vi "Example.vi"() -> ()   [LabVIEW 2013, in "Mercury iXX.lvlib"]
uses:
  <instrlib>/Mercury iXX/Mercury iXX.lvlib
  <instrlib>/Mercury iXX/Public/Controls/Unit String.ctl
  <instrlib>/Mercury iXX/Public/Libraries/Temperature/Controls/Temperature Device (Read).ctl
  <instrlib>/Mercury iXX/Public/Controls/Manufacturing Data.ctl
  <instrlib>/Mercury iXX/Public/Libraries/Temperature/Controls/Temperature Sensor Type.ctl
  <instrlib>/Mercury iXX/Public/Libraries/Temperature/Controls/Excitation Cluster.ctl
  <instrlib>/Mercury iXX/Public/Libraries/Temperature/Controls/Excitation Type.ctl
  <instrlib>/Mercury iXX/Public/Libraries/Temperature/Controls/Calibration Cluster.ctl
  <instrlib>/Mercury iXX/Public/Libraries/Temperature/Controls/Calibration Interpolation.ctl
  <instrlib>/Mercury iXX/Public/Libraries/Temperature/Controls/Loop Cluster.ctl
  <instrlib>/Mercury iXX/Public/Libraries/Temperature/Controls/Temperature Signals Cluster.ctl
  <instrlib>/Mercury iXX/Public/Libraries/Heater/Controls/Heater Device (Read).ctl
  <instrlib>/Mercury iXX/Public/Libraries/Heater/Controls/Heater Signals Cluster.ctl
  <instrlib>/Mercury iXX/Public/Libraries/Level Meter/Controls/Level Meter (Read).ctl
  <instrlib>/Mercury iXX/Public/Libraries/Level Meter/Controls/Nitrogen Configuration.ctl
  <instrlib>/Mercury iXX/Public/Libraries/Level Meter/Controls/Frequency Configuration.ctl
  <instrlib>/Mercury iXX/Public/Libraries/Level Meter/Controls/Signals.ctl
  <instrlib>/Mercury iXX/Public/Libraries/Level Meter/Controls/Helium Configuration.ctl
  <instrlib>/Mercury iXX/Public/Libraries/Level Meter/Controls/Resistance Configuration.ctl
  <instrlib>/Mercury iXX/Public/Libraries/Level Meter/Controls/Pre-Pulse.ctl
  <instrlib>/Mercury iXX/Public/Libraries/Level Meter/Controls/Pulse.ctl
  <instrlib>/Mercury iXX/Public/Libraries/Auxiliary/Controls/AUX Device (Read).ctl
  <instrlib>/Mercury iXX/Public/Libraries/Auxiliary/Controls/AUX Signals (Read).ctl
  <instrlib>/Mercury iXX/Public/Libraries/Magnet/Controls/Device (Read).ctl
  <instrlib>/Mercury iXX/Public/Libraries/Magnet/Controls/Signals (Read).ctl
  <instrlib>/Mercury iXX/Public/Libraries/Magnet/Controls/Identifier.ctl
  <instrlib>/Mercury iXX/Public/Libraries/Flow/Controls/Flow Device (Read).ctl
  <instrlib>/Mercury iXX/Public/Libraries/Flow/Controls/Flow Signals Cluster.ctl
  <instrlib>/Mercury iXX/Public/Libraries/Pressure/Controls/Pressure Device (Read).ctl
  <instrlib>/Mercury iXX/Public/Libraries/Pressure/Controls/Pressure Sensor Type.ctl
  <instrlib>/Mercury iXX/Public/Libraries/Pressure/Controls/Calibration Cluster.ctl
  <instrlib>/Mercury iXX/Public/Libraries/Pressure/Controls/Calibration Interpolation.ctl
  <instrlib>/Mercury iXX/Public/Libraries/Pressure/Controls/Loop Cluster.ctl
  <instrlib>/Mercury iXX/Public/Libraries/Pressure/Controls/Pressure Signals Cluster.ctl
  <instrlib>/Mercury iXX/Public/Controls/Comms Transport Layer.ctl
  <instrlib>/Mercury iXX/Public/Controls/ISOBus Address.ctl
  <instrlib>/Mercury iXX/Public/Libraries/System/Open/Open System.vi
  <instrlib>/Mercury iXX/Public/Libraries/Pressure/Open/Open Pressure Device.vi
  <instrlib>/Mercury iXX/Public/Libraries/Pressure/Configuration/Read/Pressure Device (Read).vi
  <instrlib>/Mercury iXX/Public/Libraries/Pressure/Configuration/Read/Nickname (Read).vi
  <instrlib>/Mercury iXX/Public/Libraries/Pressure/Signals/Read/Current (Read).vi
  <instrlib>/Mercury iXX/Public/Libraries/Pressure/Signals/Read/Voltage (Read).vi
  <instrlib>/Mercury iXX/Public/Libraries/Flow/Open/Open Flow Device.vi
  <instrlib>/Mercury iXX/Public/Libraries/Flow/Configuration/Read/Flow Device (Read).vi
  <instrlib>/Mercury iXX/Public/Libraries/Flow/Configuration/Read/Maximum Power (Read).vi
  <instrlib>/Mercury iXX/Public/Libraries/Flow/Configuration/Read/Fastcool Mode (Read).vi
  <instrlib>/Mercury iXX/Public/Libraries/Flow/Signals/Read/Current (Read).vi
  <instrlib>/Mercury iXX/Public/Libraries/Flow/Signals/Read/Voltage (Read).vi
  <instrlib>/Mercury iXX/Public/Libraries/System/Read/Catalogue (Read).vi
  <instrlib>/Mercury iXX/Public/Libraries/Auxiliary/Open/Open Auxiliary Device.vi
  <instrlib>/Mercury iXX/Public/Libraries/Auxiliary/Configuration/Read/Aux Device (Read).vi
  <instrlib>/Mercury iXX/Public/Libraries/Auxiliary/Configuration/Read/Serial Number (Read).vi
  <instrlib>/Mercury iXX/Public/Libraries/Auxiliary/Configuration/Read/Minimum Gas Flow (Read).vi
  <instrlib>/Mercury iXX/Public/Libraries/Auxiliary/Configuration/Read/Gas Flow Scaling (Read).vi
  <instrlib>/Mercury iXX/Public/Libraries/Auxiliary/Configuration/Read/Temperature Error Sensitivity (Read).vi
  <instrlib>/Mercury iXX/Public/Libraries/Auxiliary/Configuration/Read/Temperature Error Voltage Sensitivity (Read).vi
  <instrlib>/Mercury iXX/Public/Libraries/Auxiliary/Configuration/Read/Valve Gearing (Read).vi
  <instrlib>/Mercury iXX/Public/Libraries/Auxiliary/Configuration/Read/Stepper Speed (Read).vi
  <instrlib>/Mercury iXX/Public/Libraries/Auxiliary/Signals/Read/Position (Read).vi
  <instrlib>/Mercury iXX/Public/Libraries/Auxiliary/Signals/Read/Percent Open (Read).vi
  <instrlib>/Mercury iXX/Public/Libraries/Level Meter/Open/Open Level Meter Device.vi
  <instrlib>/Mercury iXX/Public/Libraries/Level Meter/Configuration/Read/Level Meter Device (Read).vi
  <instrlib>/Mercury iXX/Public/Libraries/Level Meter/Configuration/Read/Serial Number (Read).vi
  <instrlib>/Mercury iXX/Public/Libraries/Level Meter/Configuration/Read/Helium Probe Resistance (Read).vi
  <instrlib>/Mercury iXX/Public/Libraries/Level Meter/Configuration/Read/Helium Pulse Mag (Read).vi
  <instrlib>/Mercury iXX/Public/Libraries/Level Meter/Configuration/Read/Helium Pulse Duration (Read).vi
  <instrlib>/Mercury iXX/Public/Libraries/Level Meter/Configuration/Read/Nitrogen Freq at 100 (Read).vi
  <instrlib>/Mercury iXX/Public/Libraries/Level Meter/Configuration/Read/Nitrogen Pulse Count Period (Read).vi
  <instrlib>/Mercury iXX/Public/Libraries/Level Meter/Signals/Read/Probe Resistance Helium (Read).vi
  <instrlib>/Mercury iXX/Public/Libraries/Level Meter/Signals/Read/Probe Level Helium (Read).vi
  <instrlib>/Mercury iXX/Public/Libraries/Level Meter/Signals/Read/Probe Count Nitrogen (Read).vi
  <instrlib>/Mercury iXX/Public/Libraries/Level Meter/Signals/Read/Probe Level Nitrogen (Read).vi
  <instrlib>/Mercury iXX/Public/Libraries/System/Read/Display Automatic Dimming (Read).vi
  <instrlib>/Mercury iXX/Public/Libraries/System/Read/Display Automatic Dimming Time (Read).vi
  <instrlib>/Mercury iXX/Public/Libraries/System/Read/Display Brightness (Read).vi
  <instrlib>/Mercury iXX/Public/Libraries/System/Read/Date (Read).vi
  <instrlib>/Mercury iXX/Public/Libraries/System/Read/Time (Read).vi
  <instrlib>/Mercury iXX/Public/Libraries/System/Read/DateTime (Read).vi
  <instrlib>/Mercury iXX/Public/Libraries/System/Read/HVer (Read).vi
  <instrlib>/Mercury iXX/Public/Libraries/System/Read/FVer (Read).vi
  <instrlib>/Mercury iXX/Public/Libraries/System/Read/Serial Number (Read).vi
  <instrlib>/Mercury iXX/Public/Libraries/System/Read/Flash Space (Read).vi
  <instrlib>/Mercury iXX/Public/Libraries/System/Read/Mode (Read).vi
  <instrlib>/Mercury iXX/Public/Libraries/Temperature/Open/Open Temperature Device.vi
  <instrlib>/Mercury iXX/Public/Libraries/Temperature/Configuration/Read/Serial Number (Read).vi
  <instrlib>/Mercury iXX/Public/Libraries/Temperature/Configuration/Read/Nickname (Read).vi
  <instrlib>/Mercury iXX/Public/Libraries/Temperature/Configuration/Read/Excitation Magnitude (Read).vi
  <instrlib>/Mercury iXX/Public/Libraries/Temperature/Configuration/Read/Temperature Sensor (Read).vi
  <instrlib>/Mercury iXX/Public/Libraries/Temperature/Configuration/Read/Excitation Type (Read).vi
  <instrlib>/Mercury iXX/Public/Libraries/Temperature/Configuration/Read/Calibration Hot Limit (Read).vi
  <instrlib>/Mercury iXX/Public/Libraries/Temperature/Configuration/Read/Calibration Cold Limit (Read).vi
  <instrlib>/Mercury iXX/Public/Libraries/Temperature/Signals/Read/Temperature (Read).vi
  <instrlib>/Mercury iXX/Public/Libraries/Temperature/Configuration/Read/Temperature Device (Read).vi
  <instrlib>/Mercury iXX/Public/Libraries/Control Loop/Configuration/Read/Control Loop (Read).vi
  <instrlib>/Mercury iXX/Public/Libraries/Heater/Open/Open Heater Device.vi
  <instrlib>/Mercury iXX/Public/Libraries/Heater/Configuration/Read/Heater Device (Read).vi
  <instrlib>/Mercury iXX/Public/Libraries/Heater/Configuration/Read/Nickname (Read).vi
  <instrlib>/Mercury iXX/Public/Libraries/Heater/Configuration/Read/Serial Number (Read).vi
  <instrlib>/Mercury iXX/Public/Libraries/Heater/Configuration/Read/Voltage Limit (Read).vi
  <instrlib>/Mercury iXX/Public/Libraries/Heater/Configuration/Read/Nominal Resistance (Read).vi
  <instrlib>/Mercury iXX/Public/Libraries/Heater/Configuration/Read/Maximum Power (Read).vi
  <instrlib>/Mercury iXX/Public/Libraries/Heater/Signals/Read/Voltage (Read).vi
  <instrlib>/Mercury iXX/Public/Libraries/Heater/Signals/Read/Power (Read).vi
  <instrlib>/Mercury iXX/Public/Libraries/Heater/Signals/Read/Current (Read).vi
  <instrlib>/Mercury iXX/Public/Libraries/System/Set/DateTime (Set).vi
  <instrlib>/Mercury iXX/Public/Libraries/Magnet/Open/Open Magnet Device.vi
  <instrlib>/Mercury iXX/Public/Libraries/Magnet/Configuration/Read/Magnet Device (Read).vi
  <instrlib>/Mercury iXX/Public/Libraries/Magnet/Configuration/Read/Serial Number (Read).vi
  <instrlib>/Mercury iXX/Public/Libraries/Magnet/Configuration/Read/Bipolar Output (Read).vi
  <instrlib>/Mercury iXX/Public/Libraries/Magnet/Configuration/Read/Output Configuration (Read).vi
  <instrlib>/Mercury iXX/Public/Libraries/Magnet/Configuration/Read/Current Limit (Read).vi
  <instrlib>/Mercury iXX/Public/Libraries/Magnet/Configuration/Read/Current to Field Factor (Read).vi
  <instrlib>/Mercury iXX/Public/Libraries/Magnet/Configuration/Read/Switch Present (Read).vi
  <instrlib>/Mercury iXX/Public/Libraries/Magnet/Configuration/Read/Software Voltage Limit (Read).vi
  <instrlib>/Mercury iXX/Public/Libraries/Magnet/Signals/Read/Current Rate (Read).vi
  <instrlib>/Mercury iXX/Public/Libraries/Magnet/Configuration/Read/PSU Action Status (Read).vi
  <instrlib>/Mercury iXX/Public/Libraries/Flow.lvlib
  <instrlib>/Mercury iXX/Public/Libraries/Pressure.lvlib
  <instrlib>/Mercury iXX/Public/Libraries/System.lvlib
  <instrlib>/Mercury iXX/Public/Libraries/Level Meter.lvlib
  <instrlib>/Mercury iXX/Public/Libraries/Magnet.lvlib
  <instrlib>/Mercury iXX/Public/Libraries/Auxiliary.lvlib
  <instrlib>/Mercury iXX/Public/Libraries/Control Loop.lvlib
  <instrlib>/Mercury iXX/Public/Libraries/Heater.lvlib
  <instrlib>/Mercury iXX/Public/Libraries/Temperature.lvlib
panel:
  in  "Mercury Functions":T1(tab)
  in  "IPS IP Address":string="130.49.180.102"
  out "time stamp":timestamp=timestamp(3542718986 s since 1904-01-01)
  out "Free Space":i32=166152 caption="Free Space (KB)"
  out "Set Date Response":string="VALID"
  out "String":string="NORM" caption="User Mode"
  out "Date":string="2016:04:05"
  out "Time":string="11:36:26"
  out "Hardware Version":string="65"
  out "Firmware Version":string="2.2.6.20"
  out "Serial Number":string="153350063"
  out "Devices":string[](array[string])=["DB3.L1:LVL", "GRPX:PSU", "GRPY:PSU", "GRPZ:PSU", "MB1.T1:TEMP", "PSU.M1:PSU", "PSU.M2:PSU", "PSU.M3:PSU"]
  out "S/W Version(s)":string[](array[string])=["2.2.6.20\n"]
  out "Serial Number(s)":string[](array[string])=["153350063"]
  out "# of Instruments":i32=1
  out "Automatic Dimming":string="OFF"
  out "Dimming Time":string="5"
  out "Display Brightness":string="100"
  in  "ITC IP Address":string="130.49.180.102"
  out "Excitation Magnitude":dbl
  out "Sensor Type":string="DUM"
  out "Excitation Type":string="UNIP"
  out "Hot Limit":dbl=1000.0
  out "H Unit":T2="K"
  out "Cold Limit":dbl=1000.0
  out "C Unit":T2="K"
  out "Unit":T2
  out "Voltage":dbl
  out "V Unit":T2="A"
  out "Temperature":dbl
  out "T Unit":T2="K"
  out "Temperature Device Settings":T3={"Manufacturing"={"Hardware Version"="65", "Firmware Version"="2.2", "Serial Number"="153350063"}, "Temperature Sensor Type"="DUM", "Excitation"={"Excitation Type"="UNIP", "Magnitude"="0"}, "Calibration"={"Filename"="None", "Interpolation"="LIN", "Scaling Factor"="1", "Offset Factor"="0", "Hot Limit"="1000.00K", "Cold Limit"="1000.00K", "Last Calibration"="", "Reference"="Internal"}, "Control Loop"={"Heater"="", "Auxiliary"="", "Heater Auto"="", "Percentage Heat"="", "Temperature Set Point"="", "PID Auto (from file)"="", "P Value"="", "I Value"="", "D Value"="", "Auto PID Table Filename"="", "Flow Auto"="", "Target Heater Table"="", "Sweep mode"="", "Sweep Table Filename"="", "Percentage Flow"=""}, "Temperature Signals"={"Voltage"="0.0000V", "Current"="0.0000A", "Power"="N/A", "Resistance"="", "Temperature"="0.0000K", "Sensitivity"="", "Reference"=""}, "Nickname"="MB1.T1", "Status"="0"}
  out "Temp S/N":string="153350063"
  out "T Nickname":string="MB1.T1"
  out "T Loop Details":T10
  out "Heater Device Settings":T12={"Manufacturing"={"Hardware Version"="", "Firmware Version"="", "Serial Number"=""}, "Nickname"="", "Voltage Limit"="", "Nominal Resistance"="", "Maximum Power"="", "Heater Signals"={"Voltage"="", "Current"="", "Power"=""}, "Status"="DEV"}
  out "Htr C Unit":T2
  out "Htr P Unit":T2
  out "Htr V Unit":T2
  out "Htr Current":dbl
  out "Htr Power":dbl
  out "Htr Voltage":dbl
  out "Power Unit":T2
  out "Volt Unit":T2
  out "Res Unit":T2
  out "Maximum Power":dbl
  out "Htr Resistance":dbl
  out "Htr Voltage Limit":dbl
  out "Htr S/N":string="STAT:DEV:MB0.H1:N/A"
  out "Htr Nickname":string="STAT:DEV:MB0.H1:N/A"
  out "LVL Device DetailSettings":T14
  out "LVL S/N":string
  out "LVL P Magnitude":dbl=-inf caption="Pulse Magnitude (mA)"
  out "LVL P Duration":dbl=-inf caption="Pulse Duration (s)"
  out "N Freq 100%":dbl=-inf caption="Frequency at 100% (Hz)"
  out "N Pulse Period":dbl=-inf caption="Pulse Period (ms)"
  out "He Res Config":T19
  out "He Resistance":dbl=-inf caption="Resistance (Ohms)"
  out "He Level":dbl=-inf caption="Helium Level (%)"
  out "N Counter":u32 caption="Counter"
  out "N Level":dbl=-inf caption="Nitrogen Level (%)"
  out "Auxiliary Device Details":T22 {"Signals"."% Open" min=0.0 max=100.0 step=0.1 format="%.4f"; "Signals"."Position" max=20.0 step=1.0 format="%.4f"; "Speed" max=7 step=1; "Gear" max=7 step=1; "Temp V Err" min=0.0 max=20.0 step=0.1; "Temp Err" min=0.0 max=20.0 step=0.1; "Scaling Factor" min=0.0 max=99.0 step=0.1; "Min Flow" min=0.0 max=20.0 step=0.1}
  out "Aux S/N":string
  out "Min Flow":dbl=-inf caption="Minimum Gas Flow" format="%#.1f"
  out "Scaling Factor":dbl=-inf caption="Gas Flow Scaling Factor" format="%#.1f"
  out "Temp Err":dbl=-inf caption="Temperature Error Sensitivity" format="%#.1f"
  out "Temp V Err":dbl=-inf caption="Temperature Voltage Error Sensitivity" format="%#.1f"
  out "Gear":u32 caption="Valve Gearing"
  out "Speed":u32 caption="Stepper Speed"
  out "Unit 2":T2="ERR"
  out "Unit 3":T2="ERR"
  out "Unit 4":T2="ERR"
  out "Unit 5":T2="ERR"
  out "Unit 6":T2="ERR"
  out "Unit 7":T2="ERR"
  out "Position":u32
  out "% Open":dbl=-inf caption="Percentage Open (%)"
  out "Unit":T2="ERR"
  out "Unit":T2="ERR"
  out "Magnet Device Details":T24={"Manufacturing"={"Hardware Version"="65", "Firmware Version"="2.4", "Serial Number"="151250009"}, "Nickname"="PSU.M1", "Bipolar Output"="ON", "String"="NOT_FOUND", "Current Limit"=58.0, "AtoB"=1.0, "Inductance"=39.406, "Switch Present"="NOT_FOUND", "Swh Htr Current"=86.0, "SW VLIM"=9.0, "V Trans Time"=1000.0, "Magnet PSU Signals"={"Voltage"=-0.0003, "Current"=0.0002, "Current Rate"=0.0, "Field"=0.0, "Field Rate"=0.0, "Persistant Current"=0.0, "Persistant Field"=0.0, "Target Current"=0.0, "Target Field"=0.0, "Target Current Rate"=0.0, "Target Field Rate"=0.0, "Switch Heater Status (SWHT)"="NOT_FOUND", "Switch Heater Status (SWHN)"="NOT_FOUND"}, "PSU Action"="NOT_FOUND", "Status"="4000", "Level Limit"=0.0, "Temperature Limit"=0.0} {"Temperature Limit" format="%#.1f"; "Level Limit" format="%#.1f"; "V Trans Time" format="%#.1f"; "SW VLIM" format="%#.1f"; "Swh Htr Current" format="%#.1f"; "Inductance" format="%#.1f"; "AtoB" format="%#.1f"; "Current Limit" format="%#.1f"}
  out "Mag S/N":string="151250009"
  out "Bipolar Output":string="ON"
  out "Out Config":string="NOT_FOUND" caption="Output Configuration"
  out "Current Limit":dbl=58.0 caption="Current Limit (A)" format="%#.1f"
  out "AtoB":dbl=1.0 caption="Current Field Factor (A/T)" format="%#.1f"
  out "Switch Present":string="NOT_FOUND"
  out "SW VLIM":dbl=9.0 caption="Software Voltage Limit (V)" format="%#.1f"
  out "Unit 8":T2
  out "Unit 9":T2
  out "Unit 10":T2
  out "Current Rate":dbl
  out "PSU Act Stat":string="NOT_FOUND" caption="PSU Action Status"
  out "Unit 11":T2
  in  "Device Identifier":T26="PSU.M1"
  in  "Magnet?":bool=TRUE
  out "Flow Device":T27={"Manufacturing"={"Hardware Version"="", "Firmware Version"="", "Serial Number"=""}, "Nickname"="", "Voltage Limit"="", "Nominal Resistance"="", "Maximum Power"="", "Flow Signals"={"Voltage"="", "Current"="", "Power"="", "Flow"=""}, "Status"="DEV", "Fastcool Mode"=""}
  out "Maximum Power":dbl
  out "Fastcool Mode":string="STAT:DEV:DB1.F1:N/A"
  out "Current":dbl
  out "Voltage":dbl
  out "Pressure Device":T29={"Manufacturing"={"Hardware Version"="", "Firmware Version"="", "Serial Number"=""}, "Temperature Sensor Type"="", "Calibration"={"Filename"="", "Interpolation"="", "Scaling Factor"="", "Offset Factor"="", "High Limit"="", "Low Limit"="", "Last Calibration"=""}, "Control Loop"={"Heater"="", "Auxiliary"="", "Heater Auto"="", "Percentage Heat"="", "Pressure Set Point"="", "PID Auto (from file)"="", "P Value"="", "I Value"="", "D Value"="", "Auto PID Table Filename"="", "Flow Auto"="", "Target Heater Table"="", "Sweep mode"="", "Sweep Table Filename"="", "Percentage Flow"=""}, "Pressure Signals"={"Voltage"="", "Current"="", "Power"="", "Pressure"=""}, "Nickname"="", "Status"="DEV"}
  out "Nickname":string="STAT:DEV:DB6.P1:N/A"
  out "Current":dbl
  out "Voltage":dbl
  # "101, 102, 67"
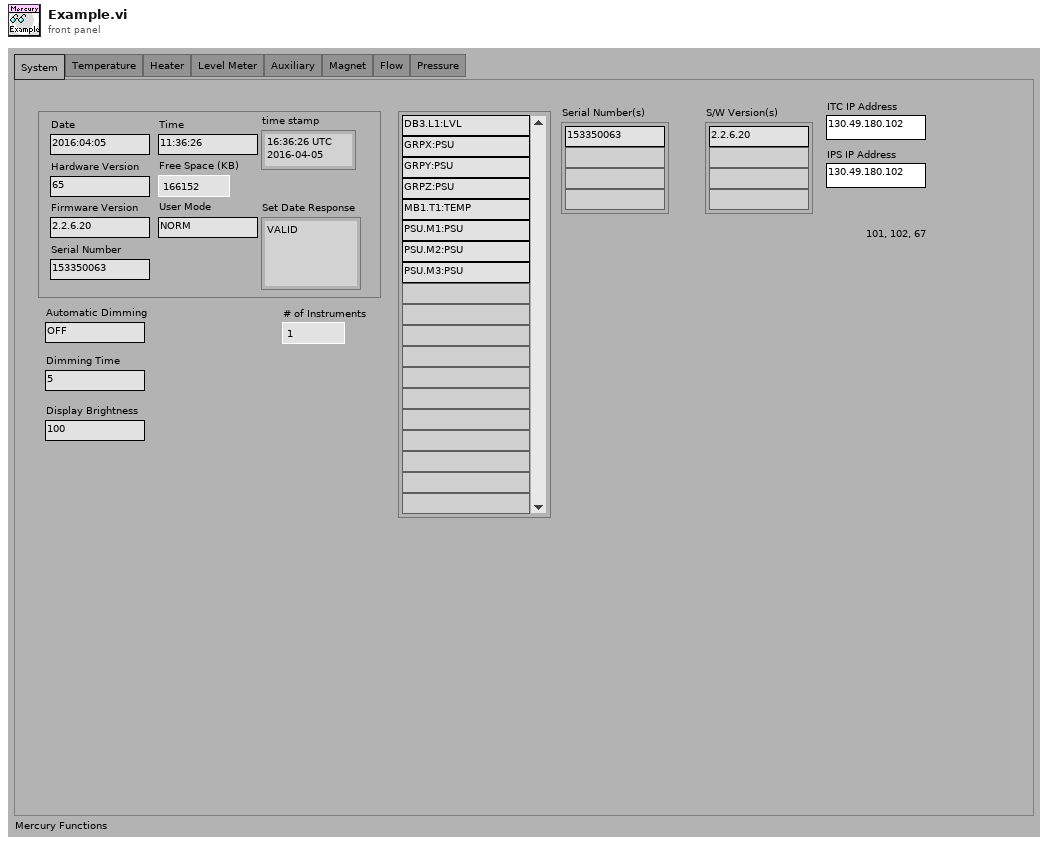
[diagram p1: front panel]
types:
  T1 = enum32{"System", "Temperature", "Heater", "Level Meter", "Auxiliary", "Magnet", "Flow", "Pressure"}
  T2 = typedef "Mercury iXX.lvlib/Unit String.ctl" = string
  T3 = typedef "Mercury iXX.lvlib/Temperature.lvlib/Temperature Device (Read).ctl" = cluster{"Manufacturing":T4, "Temperature Sensor Type":T5, "Excitation":T6, "Calibration":T8, "Control Loop":T10, "Temperature Signals":T11, "Nickname":string, "Status":string}
  T4 = typedef "Mercury iXX.lvlib/Manufacturing Data.ctl" = cluster{"Hardware Version":string, "Firmware Version":string, "Serial Number":string}
  T5 = typedef "Mercury iXX.lvlib/Temperature.lvlib/Temperature Sensor Type.ctl" = string
  T6 = typedef "Mercury iXX.lvlib/Temperature.lvlib/Excitation Cluster.ctl" = cluster{"Excitation Type":T7, "Magnitude":string}
  T7 = typedef "Mercury iXX.lvlib/Temperature.lvlib/Excitation Type.ctl" = string
  T8 = typedef "Mercury iXX.lvlib/Temperature.lvlib/Calibration Cluster.ctl" = cluster{"Filename":string, "Interpolation":T9, "Scaling Factor":string, "Offset Factor":string, "Hot Limit":string, "Cold Limit":string, "Last Calibration":string, "Reference":string}
  T9 = typedef "Mercury iXX.lvlib/Temperature.lvlib/Calibration Interpolation.ctl" = string
  T10 = typedef "Mercury iXX.lvlib/Temperature.lvlib/Loop Cluster.ctl" = cluster{"Heater":string, "Auxiliary":string, "Heater Auto":string, "Percentage Heat":string, "Temperature Set Point":string, "PID Auto (from file)":string, "P Value":string, "I Value":string, "D Value":string, "Auto PID Table Filename":string, "Flow Auto":string, "Target Heater Table":string, "Sweep mode":string, "Sweep Table Filename":string, "Percentage Flow":string}
  T11 = typedef "Mercury iXX.lvlib/Temperature.lvlib/Temperature Signals Cluster.ctl" = cluster{"Voltage":string, "Current":string, "Power":string, "Resistance":string, "Temperature":string, "Sensitivity":string, "Reference":string}
  T12 = typedef "Mercury iXX.lvlib/Heater.lvlib/Heater Device (Read).ctl" = cluster{"Manufacturing":T4, "Nickname":string, "Voltage Limit":string, "Nominal Resistance":string, "Maximum Power":string, "Heater Signals":T13, "Status":string}
  T13 = typedef "Mercury iXX.lvlib/Heater.lvlib/Heater Signals Cluster.ctl" = cluster{"Voltage":string, "Current":string, "Power":string}
  T14 = typedef "Mercury iXX.lvlib/Level Meter.lvlib/Level Meter (Read).ctl" = cluster{"Manufacturing":T4, "Nitrogen Configuration":T15, "Signals":T17, "Nickname":string, "Status":string, "Helium Configuration":T18}
  T15 = typedef "Mercury iXX.lvlib/Level Meter.lvlib/Nitrogen Configuration.ctl" = cluster{"Frequency Configuration":T16, "Pulse Period":dbl}
  T16 = typedef "Mercury iXX.lvlib/Level Meter.lvlib/Frequency Configuration.ctl" = cluster{"Freq 0%":dbl, "Freq 100%":dbl}
  T17 = typedef "Mercury iXX.lvlib/Level Meter.lvlib/Signals.ctl" = cluster{"Helium Signals":cluster{"Resistance":dbl, "Level":dbl}, "Nitrogen Signals":cluster{"Count":dbl, "Freq":dbl, "Level":dbl}}
  T18 = typedef "Mercury iXX.lvlib/Level Meter.lvlib/Helium Configuration.ctl" = cluster{"Resistance Configuration":T19, "Pre-Pulse":T20, "Pulse":T21}
  T19 = typedef "Mercury iXX.lvlib/Level Meter.lvlib/Resistance Configuration.ctl" = cluster{"Res 0%":dbl, "Res 100%":dbl}
  T20 = typedef "Mercury iXX.lvlib/Level Meter.lvlib/Pre-Pulse.ctl" = cluster{"Magnitude":dbl, "Duration":dbl}
  T21 = typedef "Mercury iXX.lvlib/Level Meter.lvlib/Pulse.ctl" = cluster{"Magnitude":dbl, "Duration":dbl, "Delay":dbl}
  T22 = typedef "Mercury iXX.lvlib/Auxiliary.lvlib/AUX Device (Read).ctl" = cluster{"Manufacturing":T4, "Min Flow":dbl, "Scaling Factor":dbl, "Temp Err":dbl, "Temp V Err":dbl, "Gear":u32, "Speed":u32, "Signals":T23, "Nickname":string, "Status":string}
  T23 = typedef "Mercury iXX.lvlib/Auxiliary.lvlib/AUX Signals (Read).ctl" = cluster{"Position":dbl, "% Open":dbl, "I0":string, "I1":string, "I2":string, "I3":string, "O0":string, "O1":string, "O2":string, "O3":string}
  T24 = typedef "Mercury iXX.lvlib/Magnet.lvlib/Device (Read).ctl" = cluster{"Manufacturing":T4, "Nickname":string, "Bipolar Output":string, "String":string, "Current Limit":dbl, "AtoB":dbl, "Inductance":dbl, "Switch Present":string, "Swh Htr Current":dbl, "SW VLIM":dbl, "V Trans Time":dbl, "Magnet PSU Signals":T25, "PSU Action":string, "Status":string, "Level Limit":dbl, "Temperature Limit":dbl}
  T25 = typedef "Mercury iXX.lvlib/Magnet.lvlib/Signals (Read).ctl" = cluster{"Voltage":dbl, "Current":dbl, "Current Rate":dbl, "Field":dbl, "Field Rate":dbl, "Persistant Current":dbl, "Persistant Field":dbl, "Target Current":dbl, "Target Field":dbl, "Target Current Rate":dbl, "Target Field Rate":dbl, "Switch Heater Status (SWHT)":string, "Switch Heater Status (SWHN)":string}
  T26 = typedef "Mercury iXX.lvlib/Magnet.lvlib/Identifier.ctl" = string
  T27 = typedef "Mercury iXX.lvlib/Flow.lvlib/Flow Device (Read).ctl" = cluster{"Manufacturing":T4, "Nickname":string, "Voltage Limit":string, "Nominal Resistance":string, "Maximum Power":string, "Flow Signals":T28, "Status":string, "Fastcool Mode":string}
  T28 = typedef "Mercury iXX.lvlib/Flow.lvlib/Flow Signals Cluster.ctl" = cluster{"Voltage":string, "Current":string, "Power":string, "Flow":string}
  T29 = typedef "Mercury iXX.lvlib/Pressure.lvlib/Pressure Device (Read).ctl" = cluster{"Manufacturing":T4, "Temperature Sensor Type":T30, "Calibration":T31, "Control Loop":T33, "Pressure Signals":T34, "Nickname":string, "Status":string}
  T30 = typedef "Mercury iXX.lvlib/Pressure.lvlib/Pressure Sensor Type.ctl" = string
  T31 = typedef "Mercury iXX.lvlib/Pressure.lvlib/Calibration Cluster.ctl" = cluster{"Filename":string, "Interpolation":T32, "Scaling Factor":string, "Offset Factor":string, "High Limit":string, "Low Limit":string, "Last Calibration":string}
  T32 = typedef "Mercury iXX.lvlib/Pressure.lvlib/Calibration Interpolation.ctl" = string
  T33 = typedef "Mercury iXX.lvlib/Pressure.lvlib/Loop Cluster.ctl" = cluster{"Heater":string, "Auxiliary":string, "Heater Auto":string, "Percentage Heat":string, "Pressure Set Point":string, "PID Auto (from file)":string, "P Value":string, "I Value":string, "D Value":string, "Auto PID Table Filename":string, "Flow Auto":string, "Target Heater Table":string, "Sweep mode":string, "Sweep Table Filename":string, "Percentage Flow":string}
  T34 = typedef "Mercury iXX.lvlib/Pressure.lvlib/Pressure Signals Cluster.ctl" = cluster{"Voltage":string, "Current":string, "Power":string, "Pressure":string}
  T35 = typedef "Mercury iXX.lvlib/ISOBus Address.ctl" = i32
  T36 = typedef "Mercury iXX.lvlib/Comms Transport Layer.ctl" = enum16{"Ethernet TCP/IP", "USB", "ISOBus - RS-232", "GPIB"}
  T37 = typedef "Mercury iXX.lvlib/Mercury Reference.ctl" = cluster{"Comms":refnum<visa-resource-name>, "Device ID":string[], "Comms Layer":T36, "Command":string, "Query reference":T38}
  T38 = typedef "Mercury iXX.lvlib/Query Dynamic Reference.ctl" = refnum<vi>
  T39 = typedef "Mercury iXX.lvlib/Magnet.lvlib/Output Configuration.ctl" = string
  T40 = typedef "Mercury iXX.lvlib/Magnet.lvlib/PSU Actions.ctl" = string
  T41 = typedef "Mercury iXX.lvlib/System.lvlib/User Mode.ctl" = string
  T42 = typedef "Mercury iXX.lvlib/Response String.ctl" = string
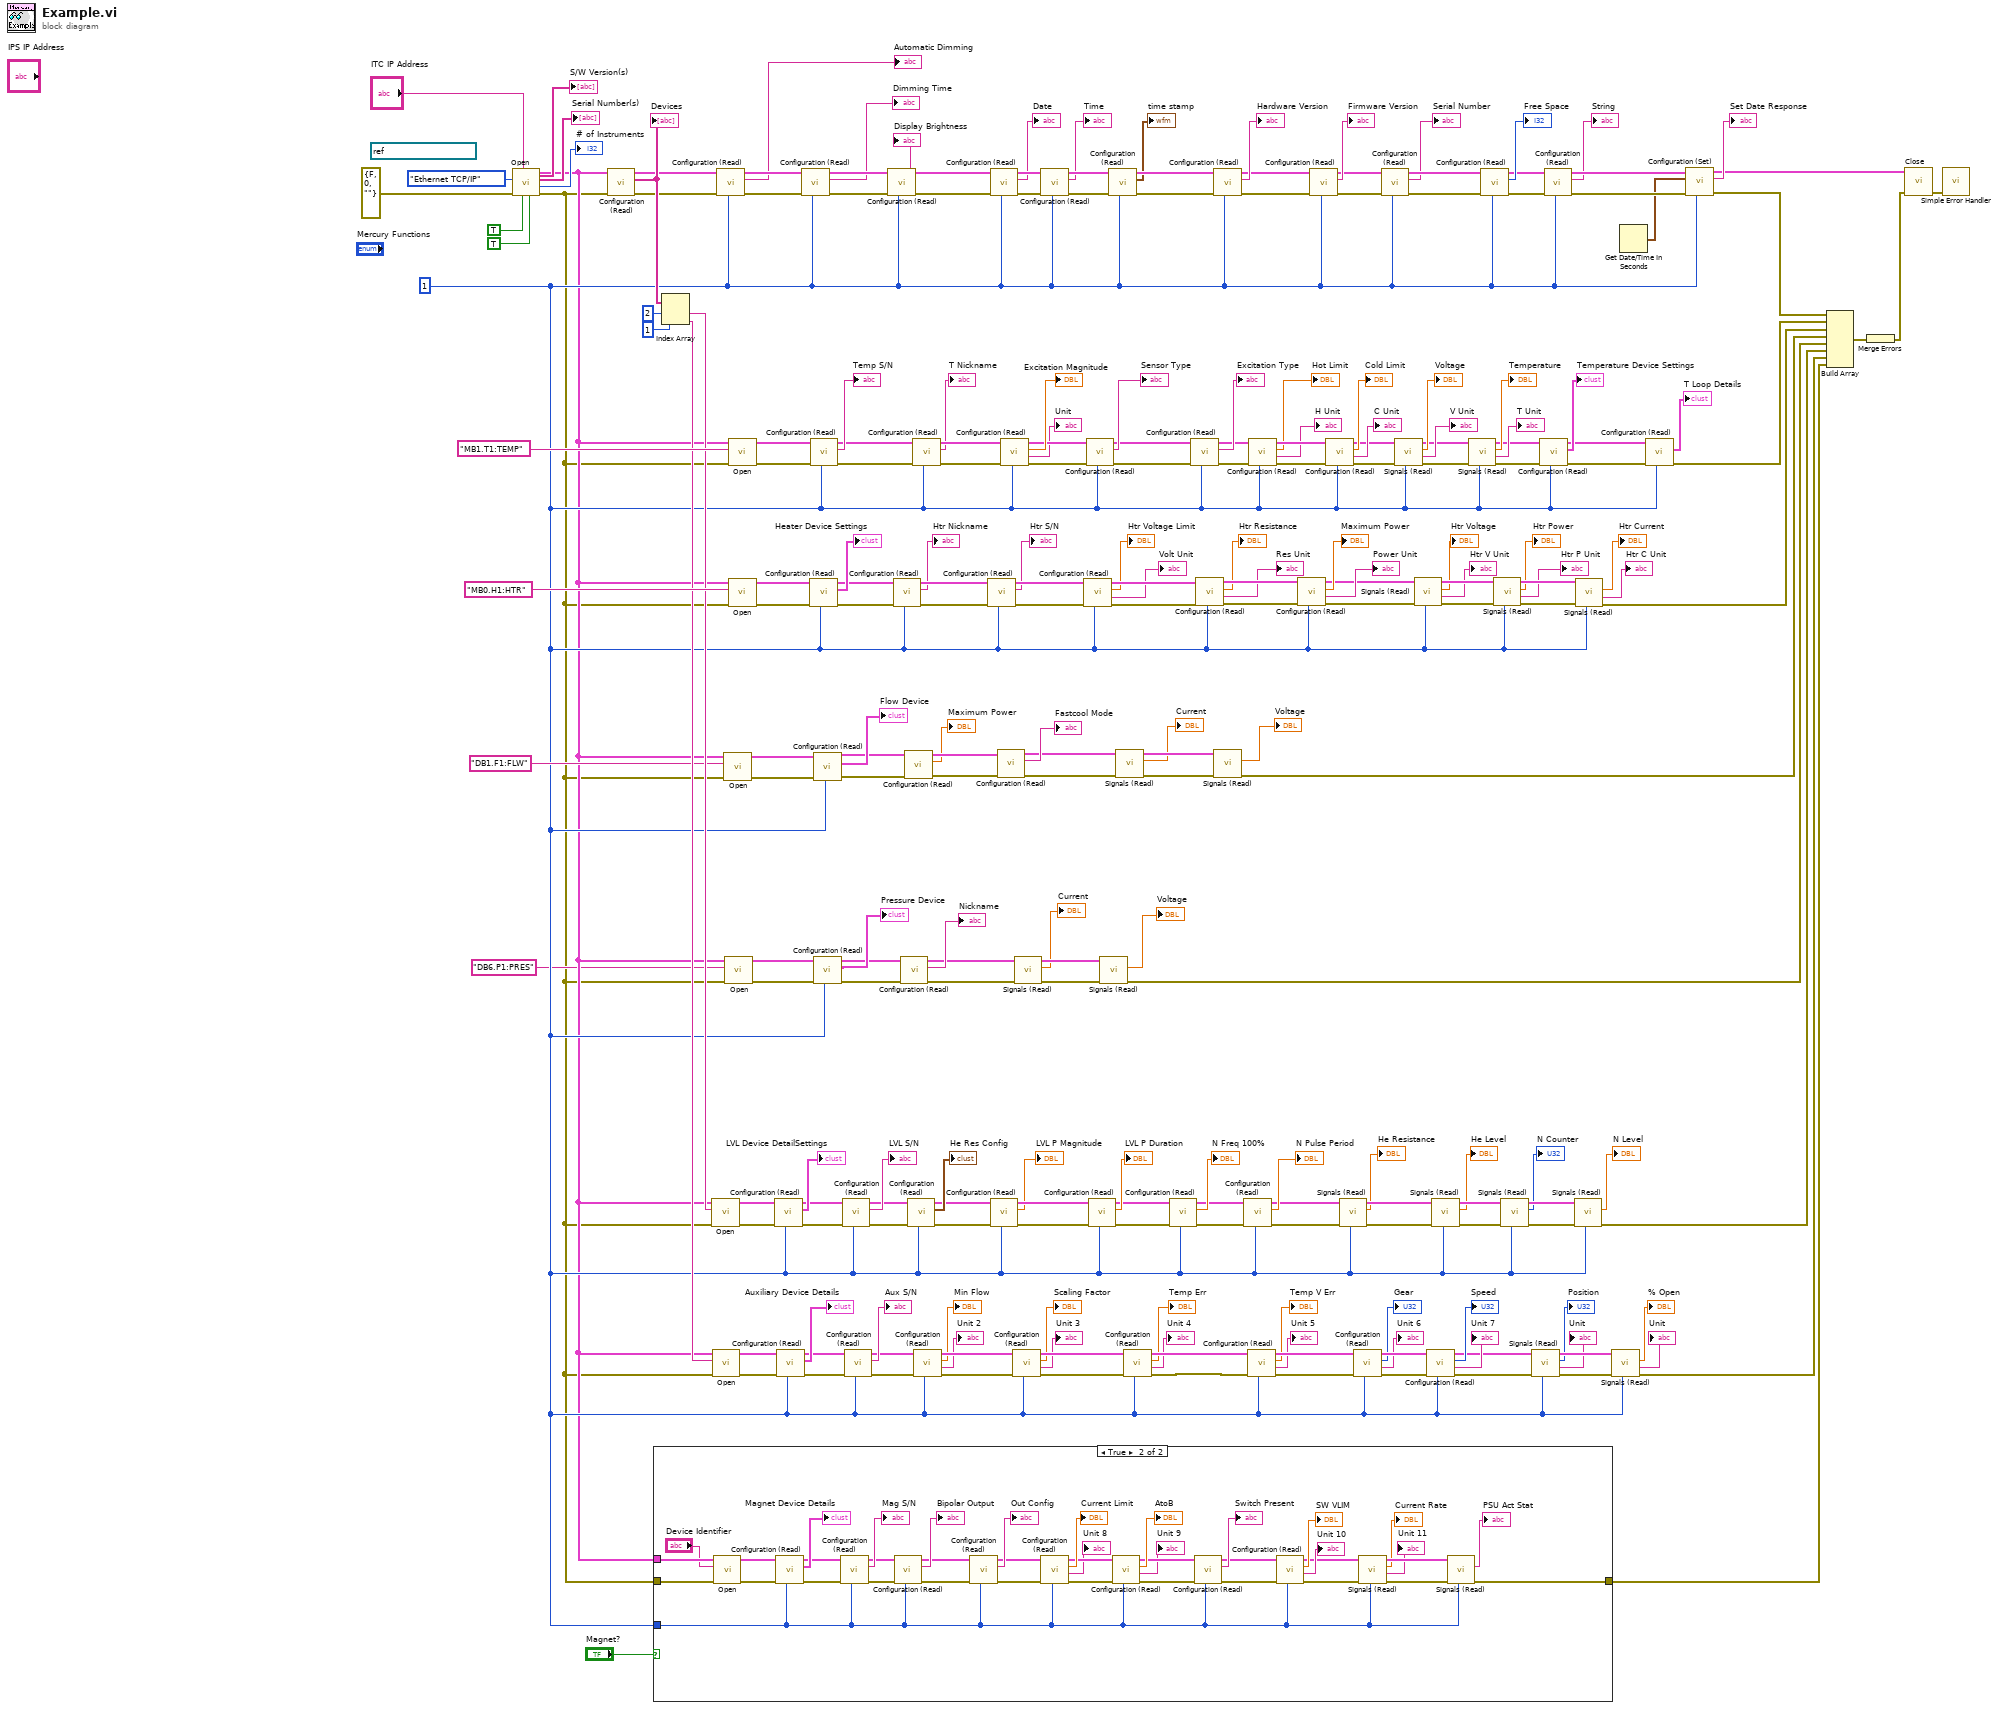
[diagram p0: block diagram]
diagram:
  w24 = T35 1 ("ISOBUS address")
  (unwired) refnum<visa-resource-name> "COM1" ("VISA resource name")
  n1 = call-poly <instrlib>:"Open.vi"("Clear Previous Connections (False)"=TRUE ("Clear Previous Connections (True)"), "ID Query (True)"=TRUE, "IP Address"="ITC IP Address", "error in (no error)"=errorcluster {"status"=FALSE, "code"=0, "source"=""}, "Comms Layer"=Comms_Transport_Layer."Ethernet TCP/IP") -> ("error out"=w21:errorcluster, "# of Instruments"=→"# of Instruments":i32, "Serial Number(s)"=→"Serial Number(s)":string[], "Mercury Reference Out"=w23:T37, "S/W Version(s)"=→"S/W Version(s)":string[])  [unwired: 2 in]
  n2 = call-poly <instrlib>:"Configuration (Read).vi"("error in"=w21, "Mercury Reference In"=w23) -> ("error out"=w41:errorcluster, "Devices"=w154:string[], "Mercury Reference Out"=w40:T37)  [unwired: 1 in, 6 out]
  "Devices" <- w154
  n3 = case shown="True" "Magnet?" {
    tunnel: w23 -> [_ w279]
    tunnel: w21 -> [w240 w278]
    tunnel: w24 -> [_ w245]
    tunnel: [w240 w247] -> w66
    frame False {
    }
    frame True {
      n4 = call-poly <instrlib>:"Open.vi"("error in (no error)"=w278, "Device Identifier"="Device Identifier", "Mercury Reference In"=w279) -> ("error out"=w276:errorcluster, "Mercury Reference Out"=w277:T37)  [unwired: 7 out]
      n5 = call-poly <instrlib>:"Configuration (Read).vi"("ISOBUS address"=w245, "error in"=w276, "Mercury Reference In"=w277) -> ("error out"=w273:errorcluster, "Magnet Device Details"=→"Magnet Device Details":T24, "Mercury Reference Out"=w274:T37)  [unwired: 6 out]
      n6 = call-poly <instrlib>:"Configuration (Read).vi"("ISOBUS address"=w245, "error in"=w273, "Mercury Reference In"=w274) -> ("error out"=w270:errorcluster, "Serial Number"=→"Mag S/N":string, "Mercury Reference Out"=w271:T37)  [unwired: 6 out]
      n7 = call-poly <instrlib>:"Configuration (Read).vi"("ISOBUS address"=w245, "error in"=w270, "Mercury Reference In"=w271) -> ("error out"=w267:errorcluster, "Bipolar Output"=→"Bipolar Output":string, "Mercury Reference Out"=w268:T37)  [unwired: 6 out]
      n8 = call-poly <instrlib>:"Configuration (Read).vi"("ISOBUS address"=w245, "error in"=w267, "Mercury Reference In"=w268) -> ("error out"=w264:errorcluster, "Out Config"=→"Out Config":T39, "Mercury Reference Out"=w265:T37)  [unwired: 6 out]
      n9 = call-poly <instrlib>:"Configuration (Read).vi"("ISOBUS address"=w245, "error in"=w264, "Mercury Reference In"=w265) -> ("error out"=w261:errorcluster, "Unit"=→"Unit 8":T2, "Current Limit"=→"Current Limit":dbl, "Mercury Reference Out"=w262:T37)  [unwired: 5 out]
      n10 = call-poly <instrlib>:"Configuration (Read).vi"("ISOBUS address"=w245, "error in"=w261, "Mercury Reference In"=w262) -> ("error out"=w258:errorcluster, "Unit"=→"Unit 9":T2, "AtoB"=→"AtoB":dbl, "Mercury Reference Out"=w259:T37)  [unwired: 5 out]
      n11 = call-poly <instrlib>:"Configuration (Read).vi"("ISOBUS address"=w245, "error in"=w258, "Mercury Reference In"=w259) -> ("error out"=w255:errorcluster, "Switch Present"=→"Switch Present":string, "Mercury Reference Out"=w256:T37)  [unwired: 6 out]
      n12 = call-poly <instrlib>:"Configuration (Read).vi"("ISOBUS address"=w245, "error in"=w255, "Mercury Reference In"=w256) -> ("error out"=w249:errorcluster, "Unit"=→"Unit 10":T2, "SW VLIM"=→"SW VLIM":dbl, "Mercury Reference Out"=w250:T37)  [unwired: 5 out]
      n13 = call-poly <instrlib>:"Signals (Read).vi"("ISOBUS address"=w245, "error in"=w249, "Mercury Reference In"=w250) -> ("error out"=w246:errorcluster, "Unit"=→"Unit 11":T2, "Current Rate"=→"Current Rate":dbl, "Mercury Reference Out"=w248:T37)  [unwired: 5 out]
      n14 = call-poly <instrlib>:"Signals (Read).vi"("ISOBUS address"=w245, "error in"=w246, "Mercury Reference In"=w248) -> ("error out"=w247:errorcluster, "PSU Act Stat"=→"PSU Act Stat":T40)  [unwired: 7 out]
    }
  }
  n15 = Index Array(array=w154, index #1=2 ("index"), index #2=1 ("index")) -> (element #1=w185:string, element #2=w184:string)
  n16 = call-poly <instrlib>:"Open.vi"("error in (no error)"=w21, "Device Identifier"=w185, "Mercury Reference In"=w23) -> ("error out"=w137:errorcluster, "Mercury Reference Out"=w138:T37)  [unwired: 7 out]
  n17 = call-poly <instrlib>:"Open.vi"("error in (no error)"=w21, "Device Identifier"=w184, "Mercury Reference In"=w23) -> ("error out"=w136:errorcluster, "Mercury Reference Out"=w135:T37)  [unwired: 7 out]
  n18 = call-poly <instrlib>:"Configuration (Read).vi"("ISOBUS address"=w24, "error in"=w41, "Mercury Reference In"=w40) -> ("error out"=w48:errorcluster, "Automatic Dimming"=→"Automatic Dimming":string, "Mercury Reference Out"=w47:T37)  [unwired: 6 out]
  n19 = call-poly <instrlib>:"Open.vi"("error in (no error)"=w21, "Device Identifier"="DB1.F1:FLW", "Mercury Reference In"=w23) -> ("error out"=w35:errorcluster, "Mercury Reference Out"=w36:T37)  [unwired: 7 out]
  n20 = call-poly <instrlib>:"Open.vi"("error in (no error)"=w21, "Device Identifier"="DB6.P1:PRES", "Mercury Reference In"=w23) -> ("error out"=w20:errorcluster, "Mercury Reference Out"=w19:T37)  [unwired: 7 out]
  n21 = call-poly <instrlib>:"Open.vi"("error in (no error)"=w21, "Device Identifier"="MB1.T1:TEMP", "Mercury Reference In"=w23) -> ("error out"=w52:errorcluster, "Mercury Reference Out"=w51:T37)  [unwired: 7 out]
  n22 = call-poly <instrlib>:"Open.vi"("error in (no error)"=w21, "Device Identifier"="MB0.H1:HTR", "Mercury Reference In"=w23) -> ("error out"=w188:errorcluster, "Mercury Reference Out"=w189:T37)  [unwired: 7 out]
  n23 = call-poly <instrlib>:"Configuration (Read).vi"("ISOBUS address"=w24, "error in"=w137, "Mercury Reference In"=w138) -> ("error out"=w129:errorcluster, "LVL Device Settings"=→"LVL Device DetailSettings":T14, "Mercury Reference Out"=w132:T37)  [unwired: 6 out]
  n24 = call-poly <instrlib>:"Configuration (Read).vi"("ISOBUS address"=w24, "error in"=w136, "Mercury Reference In"=w135) -> ("error out"=w113:errorcluster, "Auxiliary Device Details"=→"Auxiliary Device Details":T22, "Mercury Reference Out"=w114:T37)  [unwired: 6 out]
  n25 = call-poly <instrlib>:"Configuration (Read).vi"("ISOBUS address"=w24, "error in"=w48, "Mercury Reference In"=w47) -> ("error out"=w45:errorcluster, "Dimming Time"=→"Dimming Time":string, "Mercury Reference Out"=w46:T37)  [unwired: 6 out]
  n26 = call-poly <instrlib>:"Configuration (Read).vi"("ISOBUS address"=w24, "error in"=w188, "Mercury Reference In"=w189) -> ("error out"=w152:errorcluster, "Device Details"=→"Heater Device Settings":T12, "Mercury Reference Out"=w153:T37)  [unwired: 6 out]
  n27 = call-poly <instrlib>:"Configuration (Read).vi"("ISOBUS address"=w24, "error in"=w52, "Mercury Reference In"=w51) -> ("error out"=w221:errorcluster, "Serial Number"=→"Temp S/N":string, "Mercury Reference Out"=w222:T37)  [unwired: 6 out]
  n28 = call-poly <instrlib>:"Configuration (Read).vi"("ISOBUS address"=w24, "error in"=w35, "Mercury Reference In"=w36) -> ("error out"=w32:errorcluster, "Device Details"=→"Flow Device":T27, "Mercury Reference Out"=w31:T37)  [unwired: 6 out]
  n29 = call-poly <instrlib>:"Configuration (Read).vi"("ISOBUS address"=w24, "error in"=w20, "Mercury Reference In"=w19) -> ("error out"=w18:errorcluster, "Device Details"=→"Pressure Device":T29, "Mercury Reference Out"=w17:T37)  [unwired: 6 out]
  n30 = call-poly <instrlib>:"Configuration (Read).vi"("ISOBUS address"=w24, "error in"=w129, "Mercury Reference In"=w132) -> ("error out"=w128:errorcluster, "Serial Number"=→"LVL S/N":string, "Mercury Reference Out"=w130:T37)  [unwired: 6 out]
  n31 = call-poly <instrlib>:"Configuration (Read).vi"("ISOBUS address"=w24, "error in"=w113, "Mercury Reference In"=w114) -> ("error out"=w110:errorcluster, "Serial Number"=→"Aux S/N":string, "Mercury Reference Out"=w111:T37)  [unwired: 6 out]
  n32 = call-poly <instrlib>:"Configuration (Read).vi"("ISOBUS address"=w24, "error in"=w45, "Mercury Reference In"=w46) -> ("error out"=w39:errorcluster, "Display Brightness"=→"Display Brightness":string, "Mercury Reference Out"=w38:T37)  [unwired: 6 out]
  n33 = call-poly <instrlib>:"Configuration (Read).vi"("ISOBUS address"=w24, "error in"=w152, "Mercury Reference In"=w153) -> ("error out"=w150:errorcluster, "Nickname"=→"Htr Nickname":string, "Mercury Reference Out"=w151:T37)  [unwired: 6 out]
  n34 = call-poly <instrlib>:"Configuration (Read).vi"("error in"=w18, "Mercury Reference In"=w17) -> ("error out"=w13:errorcluster, "Nickname"=→"Nickname":string, "Mercury Reference Out"=w11:T37)  [unwired: 1 in, 6 out]
  n35 = call-poly <instrlib>:"Configuration (Read).vi"("error in"=w32, "Mercury Reference In"=w31) -> ("error out"=w33:errorcluster, "Maximum Power"=→"Maximum Power":dbl, "Mercury Reference Out"=w30:T37)  [unwired: 1 in, 6 out]
  n36 = call-poly <instrlib>:"Configuration (Read).vi"("ISOBUS address"=w24, "error in"=w128, "Mercury Reference In"=w130) -> ("error out"=w125:errorcluster, "Resistance Configuration"=→"He Res Config":T19, "Mercury Reference Out"=w126:T37)  [unwired: 6 out]
  n37 = call-poly <instrlib>:"Configuration (Read).vi"("ISOBUS address"=w24, "error in"=w221, "Mercury Reference In"=w222) -> ("error out"=w219:errorcluster, "Nickname"=→"T Nickname":string, "Mercury Reference Out"=w220:T37)  [unwired: 6 out]
  n38 = call-poly <instrlib>:"Configuration (Read).vi"("ISOBUS address"=w24, "error in"=w110, "Mercury Reference In"=w111) -> ("error out"=w108:errorcluster, "Unit"=→"Unit 2":T2, "Min Flow"=→"Min Flow":dbl, "Mercury Reference Out"=w109:T37)  [unwired: 5 out]
  n39 = call-poly <instrlib>:"Configuration (Read).vi"("ISOBUS address"=w24, "error in"=w150, "Mercury Reference In"=w151) -> ("error out"=w182:errorcluster, "Serial Number"=→"Htr S/N":string, "Mercury Reference Out"=w183:T37)  [unwired: 6 out]
  n40 = call-poly <instrlib>:"Configuration (Read).vi"("ISOBUS address"=w24, "error in"=w39, "Mercury Reference In"=w38) -> ("error out"=w238:errorcluster, "Date"=→"Date":string, "Mercury Reference Out"=w239:T37)  [unwired: 6 out]
  n41 = call-poly <instrlib>:"Configuration (Read).vi"("ISOBUS address"=w24, "error in"=w125, "Mercury Reference In"=w126) -> ("error out"=w123:errorcluster, "Magnitude"=→"LVL P Magnitude":dbl, "Mercury Reference Out"=w124:T37)  [unwired: 6 out]
  n42 = call-poly <instrlib>:"Configuration (Read).vi"("error in"=w33, "Mercury Reference In"=w30) -> ("error out"=w6:errorcluster, "Fastcool Mode"=→"Fastcool Mode":string, "Mercury Reference Out"=w5:T37)  [unwired: 1 in, 6 out]
  n43 = call-poly <instrlib>:"Configuration (Read).vi"("ISOBUS address"=w24, "error in"=w219, "Mercury Reference In"=w220) -> ("error out"=w216:errorcluster, "Unit"=→"Unit":T2, "Excitation Magnitude"=→"Excitation Magnitude":dbl, "Mercury Reference Out"=w217:T37)  [unwired: 5 out]
  n44 = call-poly <instrlib>:"Configuration (Read).vi"("ISOBUS address"=w24, "error in"=w108, "Mercury Reference In"=w109) -> ("error out"=w106:errorcluster, "Unit"=→"Unit 3":T2, "Scaling Factor"=→"Scaling Factor":dbl, "Mercury Reference Out"=w107:T37)  [unwired: 5 out]
  n45 = call-poly <instrlib>:"Signals (Read).vi"("error in"=w13, "Mercury Reference In"=w11) -> ("error out"=w15:errorcluster, "Current"=→"Current":dbl, "Mercury Reference Out"=w14:T37)  [unwired: 1 in, 6 out]
  n46 = call-poly <instrlib>:"Configuration (Read).vi"("ISOBUS address"=w24, "error in"=w238, "Mercury Reference In"=w239) -> ("error out"=w236:errorcluster, "Time"=→"Time":string, "Mercury Reference Out"=w237:T37)  [unwired: 6 out]
  n47 = call-poly <instrlib>:"Configuration (Read).vi"("ISOBUS address"=w24, "error in"=w182, "Mercury Reference In"=w183) -> ("error out"=w181:errorcluster, "Unit"=→"Volt Unit":T2, "Voltage Limit"=→"Htr Voltage Limit":dbl, "Mercury Reference Out"=w178:T37)  [unwired: 5 out]
  n48 = call-poly <instrlib>:"Configuration (Read).vi"("ISOBUS address"=w24, "error in"=w216, "Mercury Reference In"=w217) -> ("error out"=w213:errorcluster, "Sensor Type"=→"Sensor Type":T5, "Mercury Reference Out"=w214:T37)  [unwired: 6 out]
  n49 = call-poly <instrlib>:"Configuration (Read).vi"("ISOBUS address"=w24, "error in"=w123, "Mercury Reference In"=w124) -> ("error out"=w119:errorcluster, "Duration"=→"LVL P Duration":dbl, "Mercury Reference Out"=w120:T37)  [unwired: 6 out]
  n50 = call-poly <instrlib>:"Signals (Read).vi"("error in"=w15, "Mercury Reference In"=w14) -> ("error out"=w12:errorcluster, "Voltage"=→"Voltage":dbl)  [unwired: 1 in, 7 out]
  n51 = call-poly <instrlib>:"Configuration (Read).vi"("ISOBUS address"=w24, "error in"=w236, "Mercury Reference In"=w237) -> ("error out"=w234:errorcluster, "time stamp"=→"time stamp":timestamp, "Mercury Reference Out"=w235:T37)  [unwired: 6 out]
  n52 = call-poly <instrlib>:"Signals (Read).vi"("error in"=w6, "Mercury Reference In"=w5) -> ("error out"=w8:errorcluster, "Current"=→"Current":dbl, "Mercury Reference Out"=w7:T37)  [unwired: 1 in, 6 out]
  n53 = call-poly <instrlib>:"Configuration (Read).vi"("ISOBUS address"=w24, "error in"=w106, "Mercury Reference In"=w107) -> ("error out"=w104:errorcluster, "Unit"=→"Unit 4":T2, "Temp Err"=→"Temp Err":dbl, "Mercury Reference Out"=w105:T37)  [unwired: 5 out]
  n54 = call-poly <instrlib>:"Configuration (Read).vi"("ISOBUS address"=w24, "error in"=w119, "Mercury Reference In"=w120) -> ("error out"=w116:errorcluster, "Freq 100%"=→"N Freq 100%":dbl, "Mercury Reference Out"=w117:T37)  [unwired: 6 out]
  n55 = call-poly <instrlib>:"Configuration (Read).vi"("ISOBUS address"=w24, "error in"=w213, "Mercury Reference In"=w214) -> ("error out"=w211:errorcluster, "Excitation Type"=→"Excitation Type":T7, "Mercury Reference Out"=w210:T37)  [unwired: 6 out]
  n56 = call-poly <instrlib>:"Configuration (Read).vi"("ISOBUS address"=w24, "error in"=w181, "Mercury Reference In"=w178) -> ("error out"=w180:errorcluster, "Unit"=→"Res Unit":T2, "Nominal Resistance"=→"Htr Resistance":dbl, "Mercury Reference Out"=w179:T37)  [unwired: 5 out]
  n57 = call-poly <instrlib>:"Configuration (Read).vi"("ISOBUS address"=w24, "error in"=w234, "Mercury Reference In"=w235) -> ("error out"=w53:errorcluster, "Hardware Version"=→"Hardware Version":string, "Mercury Reference Out"=w54:T37)  [unwired: 6 out]
  n58 = call-poly <instrlib>:"Signals (Read).vi"("error in"=w8, "Mercury Reference In"=w7) -> ("error out"=w4:errorcluster, "Voltage"=→"Voltage":dbl)  [unwired: 1 in, 7 out]
  n59 = call-poly <instrlib>:"Configuration (Read).vi"("ISOBUS address"=w24, "error in"=w116, "Mercury Reference In"=w117) -> ("error out"=w78:errorcluster, "Pulse Period"=→"N Pulse Period":dbl, "Mercury Reference Out"=w79:T37)  [unwired: 6 out]
  n60 = call-poly <instrlib>:"Configuration (Read).vi"("ISOBUS address"=w24, "error in"=w104, "Mercury Reference In"=w105) -> ("error out"=w102:errorcluster, "Unit"=→"Unit 5":T2, "Temp V Err"=→"Temp V Err":dbl, "Mercury Reference Out"=w103:T37)  [unwired: 5 out]
  n61 = call-poly <instrlib>:"Configuration (Read).vi"("ISOBUS address"=w24, "error in"=w211, "Mercury Reference In"=w210) -> ("error out"=w209:errorcluster, "Unit"=→"H Unit":T2, "Hot Limit"=→"Hot Limit":dbl, "Mercury Reference Out"=w208:T37)  [unwired: 5 out]
  n62 = call-poly <instrlib>:"Configuration (Read).vi"("ISOBUS address"=w24, "error in"=w180, "Mercury Reference In"=w179) -> ("error out"=w170:errorcluster, "Unit"=→"Power Unit":T2, "Maximum Power"=→"Maximum Power":dbl, "Mercury Reference Out"=w171:T37)  [unwired: 5 out]
  n63 = call-poly <instrlib>:"Configuration (Read).vi"("ISOBUS address"=w24, "error in"=w53, "Mercury Reference In"=w54) -> ("error out"=w55:errorcluster, "Firmware Version"=→"Firmware Version":string, "Mercury Reference Out"=w56:T37)  [unwired: 6 out]
  n64 = call-poly <instrlib>:"Configuration (Read).vi"("ISOBUS address"=w24, "error in"=w209, "Mercury Reference In"=w208) -> ("error out"=w201:errorcluster, "Unit"=→"C Unit":T2, "Cold Limit"=→"Cold Limit":dbl, "Mercury Reference Out"=w202:T37)  [unwired: 5 out]
  n65 = call-poly <instrlib>:"Signals (Read).vi"("ISOBUS address"=w24, "error in"=w78, "Mercury Reference In"=w79) -> ("error out"=w76:errorcluster, "Resistance"=→"He Resistance":dbl, "Mercury Reference Out"=w77:T37)  [unwired: 6 out]
  n66 = call-poly <instrlib>:"Configuration (Read).vi"("ISOBUS address"=w24, "error in"=w102, "Mercury Reference In"=w103) -> ("error out"=w100:errorcluster, "Unit"=→"Unit 6":T2, "Gear"=→"Gear":u32, "Mercury Reference Out"=w101:T37)  [unwired: 5 out]
  n67 = call-poly <instrlib>:"Configuration (Read).vi"("ISOBUS address"=w24, "error in"=w55, "Mercury Reference In"=w56) -> ("error out"=w232:errorcluster, "Serial Number"=→"Serial Number":string, "Mercury Reference Out"=w233:T37)  [unwired: 6 out]
  n68 = call-poly <instrlib>:"Signals (Read).vi"("ISOBUS address"=w24, "error in"=w201, "Mercury Reference In"=w202) -> ("error out"=w197:errorcluster, "Unit"=→"V Unit":T2, "Current"=→"Voltage":dbl, "Mercury Reference Out"=w198:T37)  [unwired: 5 out]
  n69 = call-poly <instrlib>:"Signals (Read).vi"("ISOBUS address"=w24, "error in"=w170, "Mercury Reference In"=w171) -> ("error out"=w168:errorcluster, "Unit"=→"Htr V Unit":T2, "Voltage"=→"Htr Voltage":dbl, "Mercury Reference Out"=w169:T37)  [unwired: 5 out]
  n70 = call-poly <instrlib>:"Configuration (Read).vi"("ISOBUS address"=w24, "error in"=w100, "Mercury Reference In"=w101) -> ("error out"=w86:errorcluster, "Unit"=→"Unit 7":T2, "Speed"=→"Speed":u32, "Mercury Reference Out"=w87:T37)  [unwired: 5 out]
  n71 = call-poly <instrlib>:"Signals (Read).vi"("ISOBUS address"=w24, "error in"=w76, "Mercury Reference In"=w77) -> ("error out"=w74:errorcluster, "Level"=→"He Level":dbl, "Mercury Reference Out"=w75:T37)  [unwired: 6 out]
  n72 = call-poly <instrlib>:"Signals (Read).vi"("ISOBUS address"=w24, "error in"=w197, "Mercury Reference In"=w198) -> ("error out"=w196:errorcluster, "Unit"=→"T Unit":T2, "Temperature"=→"Temperature":dbl, "Mercury Reference Out"=w190:T37)  [unwired: 5 out]
  n73 = call-poly <instrlib>:"Configuration (Read).vi"("ISOBUS address"=w24, "error in"=w232, "Mercury Reference In"=w233) -> ("error out"=w155:errorcluster, "Free Space"=→"Free Space":i32, "Mercury Reference Out"=w156:T37)  [unwired: 6 out]
  n74 = call-poly <instrlib>:"Signals (Read).vi"("ISOBUS address"=w24, "error in"=w168, "Mercury Reference In"=w169) -> ("error out"=w166:errorcluster, "Unit"=→"Htr P Unit":T2, "Power"=→"Htr Power":dbl, "Mercury Reference Out"=w167:T37)  [unwired: 5 out]
  n75 = call-poly <instrlib>:"Signals (Read).vi"("ISOBUS address"=w24, "error in"=w74, "Mercury Reference In"=w75) -> ("error out"=w72:errorcluster, "Counter"=→"N Counter":u32, "Mercury Reference Out"=w73:T37)  [unwired: 6 out]
  n76 = call-poly <instrlib>:"Signals (Read).vi"("ISOBUS address"=w24, "error in"=w86, "Mercury Reference In"=w87) -> ("error out"=w84:errorcluster, "Unit"=→"Unit":T2, "Position"=→"Position":u32, "Mercury Reference Out"=w85:T37)  [unwired: 5 out]
  n77 = call-poly <instrlib>:"Configuration (Read).vi"("ISOBUS address"=w24, "error in"=w196, "Mercury Reference In"=w190) -> ("error out"=w140:errorcluster, "Device Details"=→"Temperature Device Settings":T3, "Mercury Reference Out"=w142:T37)  [unwired: 6 out]
  n78 = call-poly <instrlib>:"Configuration (Read).vi"("ISOBUS address"=w24, "error in"=w155, "Mercury Reference In"=w156) -> ("error out"=w227:errorcluster, "Mode"=→"String":T41, "Mercury Reference Out"=w226:T37)  [unwired: 6 out]
  n79 = call-poly <instrlib>:"Signals (Read).vi"("ISOBUS address"=w24, "error in"=w72, "Mercury Reference In"=w73) -> ("error out"=w26:errorcluster, "Level"=→"N Level":dbl)  [unwired: 7 out]
  n80 = call-poly <instrlib>:"Signals (Read).vi"("ISOBUS address"=w24, "error in"=w166, "Mercury Reference In"=w167) -> ("error out"=w165:errorcluster, "Unit"=→"Htr C Unit":T2, "Current"=→"Htr Current":dbl)  [unwired: 6 out]
  n81 = call-poly <instrlib>:"Signals (Read).vi"("ISOBUS address"=w24, "error in"=w84, "Mercury Reference In"=w85) -> ("error out"=w27:errorcluster, "Unit"=→"Unit":T2, "% Open"=→"% Open":dbl)  [unwired: 6 out]
  n82 = Get Date/Time In Seconds() -> (seconds since 1Jan1904=w57:timestamp)
  n83 = call-poly <instrlib>:"Configuration (Read).vi"("ISOBUS address"=w24, "error in"=w140, "Mercury Reference In"=w142) -> ("error out"=w141:errorcluster, "Loop Details"=→"T Loop Details":T10)  [unwired: 7 out]
  n84 = call-poly <instrlib>:"Configuration (Set).vi"("ISOBUS address"=w24, "error in"=w227, "time stamp"=w57, "Mercury Reference In"=w226) -> ("error out"=w50:errorcluster, "Response"=→"Set Date Response":T42, "Mercury Reference Out"=w49:T37)  [unwired: 5 out]
  n85 = Build Array(w50, w141, w165, w4, w12, w26, w27, w66) -> (w1:errorcluster[])
  n86 = Merge Errors(w1) -> (w191:errorcluster)
  n87 = call <instrlib>:"Close.vi"("error in (no error)"=w191, "Mercury Reference"=w49) -> ("error out"=w60:errorcluster)  [unwired: 9 out]
  n88 = call <vilib>:"Simple Error Handler.vi"("error in (no error)"=w60) -> ()  [unwired: 1 in, 8 out]
